vi "LabVIEW调用多模态大模型.vi"() -> ()   [LabVIEW 2023, in "LabVIEW LLM.lvlib"]
uses:
  LabVIEW LLM.lvlib
  openai_complex_message.ctl
  chat-role.ctl
  complex content.ctl
  chat-completion complex req.ctl
  <vilib>/Utility/error.llb/Trim Whitespace One-Sided.vi
  labview-ai-share/LabVIEW AI Base.lvlib
  <vilib>/JDP Science/JDP Science Common Utilities/Base64/Base64 Support.lvlib
panel:
  in  "Select Image":bool
  out "Base64 Encoded":string
  out "图片":picture
  in  "API Key":string="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"
  in  "system prompt":string caption="System提示词"
  in  "temperature (default: 0.8)":dbl=0.8 format="%.1f"
  in  "max tokens (default: 4096)":u32=4096
  in  "Clear":bool
  in  "model URL":string="https://openrouter.ai/api/v1"
  in  "Send":bool
  in  "Input":string="图片中的模块是什么型号？它有几个测量通道？能测量什么类型的信号？"
  in  "选择本地模型":string(combo)="qwen/qwen2.5-vl-3b-instruct:free"
  out "error out":errorcluster
  in  "STOP":bool
  out "对话":string
  # "LabVIEW调用多模态大模型"
  # "参数"
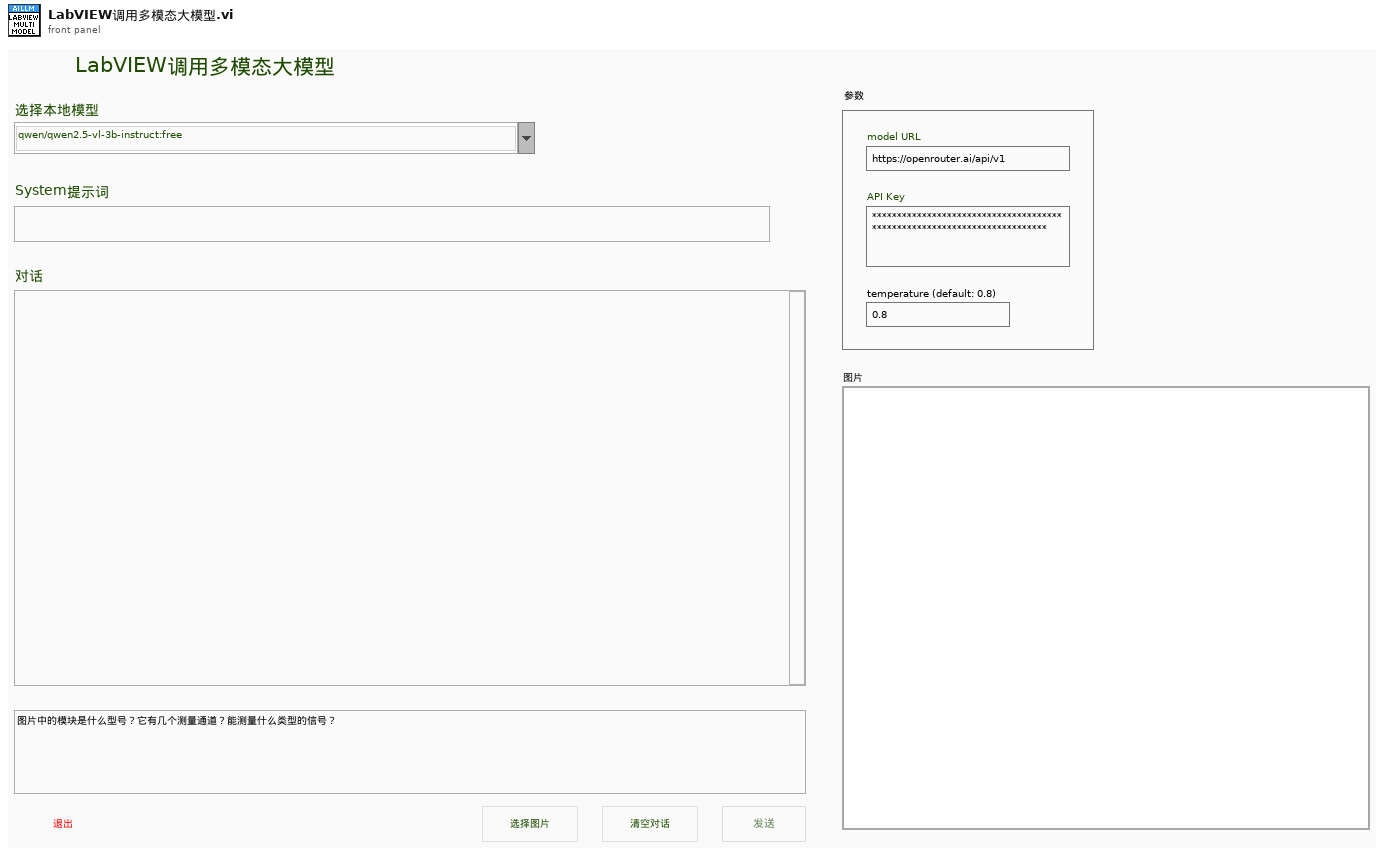
[diagram p1: front panel]
types:
  T1 = enum8{"Enabled", "Disabled", "Disabled and Grayed Out"}
  T2 = typedef "LabVIEW LLM.lvlib/openai_complex_message.ctl" = cluster{"role":T3, "content":T4[]}
  T3 = typedef "LabVIEW LLM.lvlib/chat-role.ctl" = enum16{"system", "user", "assistant"}
  T4 = typedef "LabVIEW LLM.lvlib/complex content.ctl" = cluster{"type":string, "text":string, "image_url":cluster{"url":string}}
  T5 = typedef "LabVIEWHTTPClient.lvlib/ClientHandle.ctl" = refnum<k1>
  T6 = typedef "LabVIEW LLM.lvlib/chat-completion complex req.ctl" = cluster{"model":string, "messages":T2[], "max_tokens":u32, "temperature":dbl, "stream":bool}
  T7 = typedef "LVBoundsTypeDef.ctl" = cluster{"Width":u32, "Height":u32}
  T8 = typedef "imagedata.ctl" = cluster{"image type":i32, "image depth":i32, "image":u8[], "mask":u8[], "colors":u32[], "Rectangle":cluster{"left":i16, "top":i16, "right":i16, "bottom":i16}}
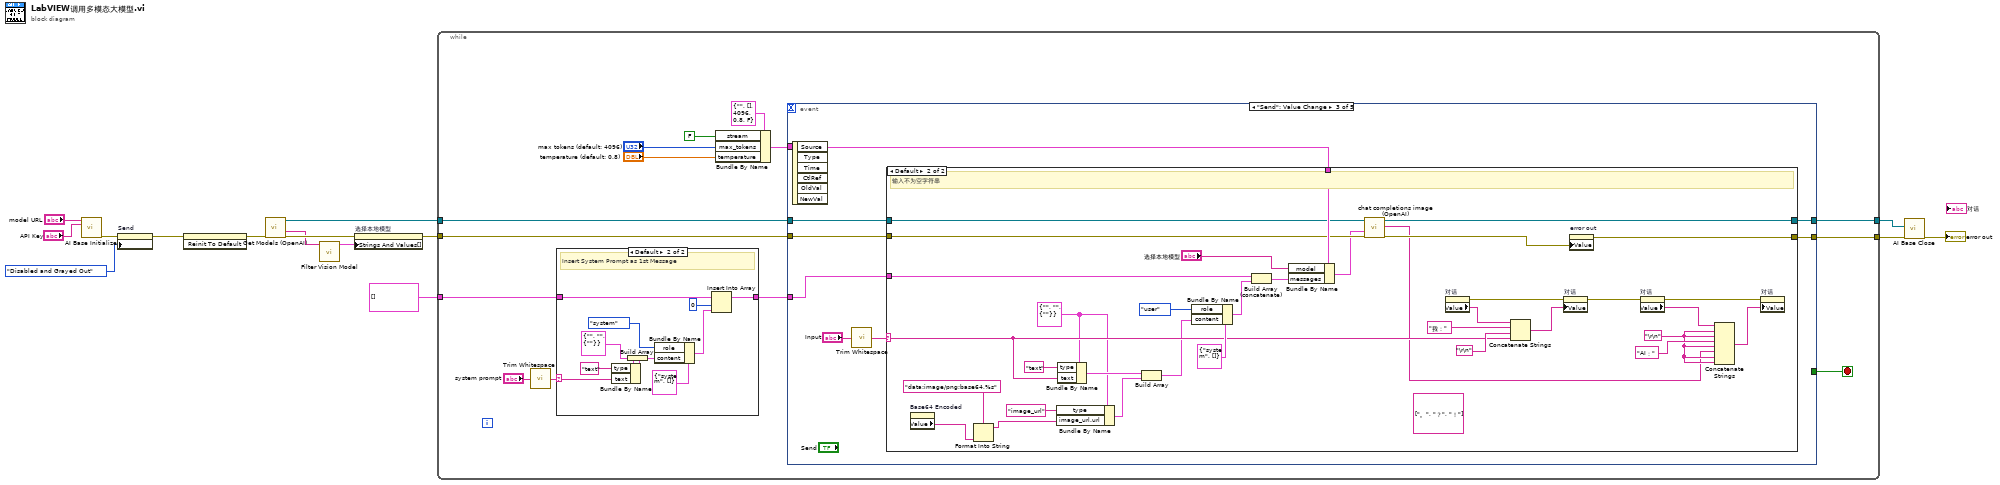
[diagram p0: block diagram]
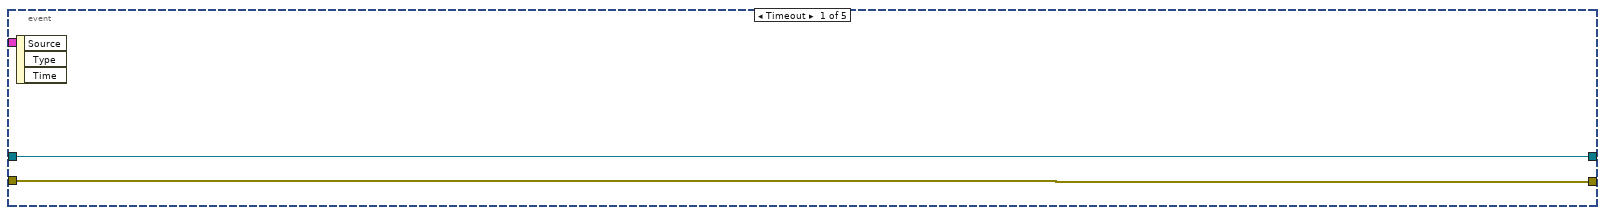
[diagram p3: hidden frame]
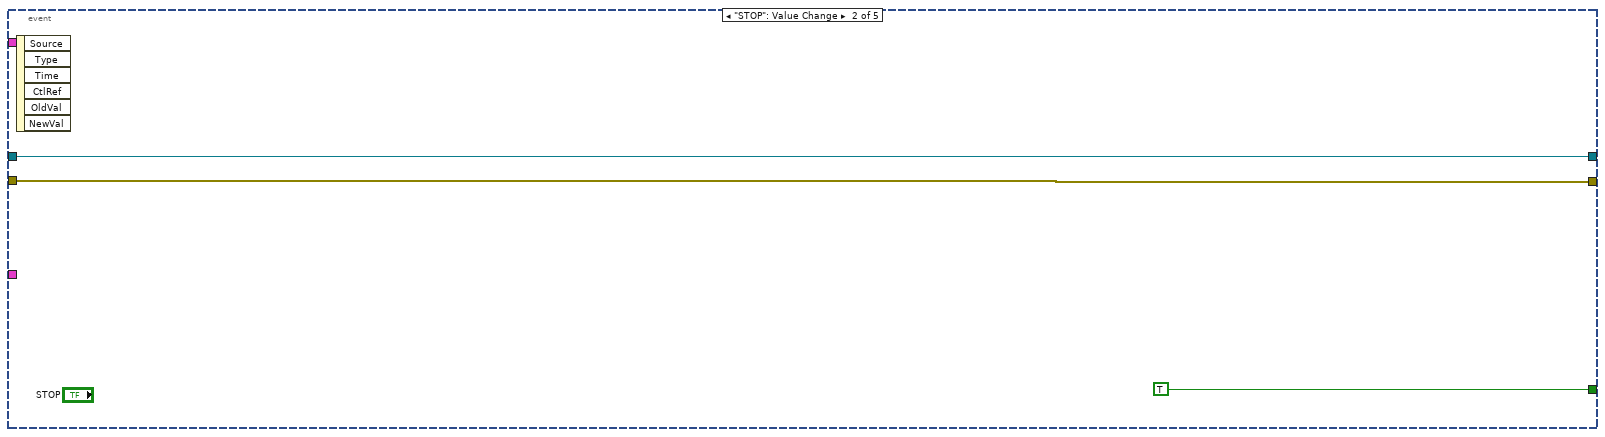
[diagram p4: hidden frame]
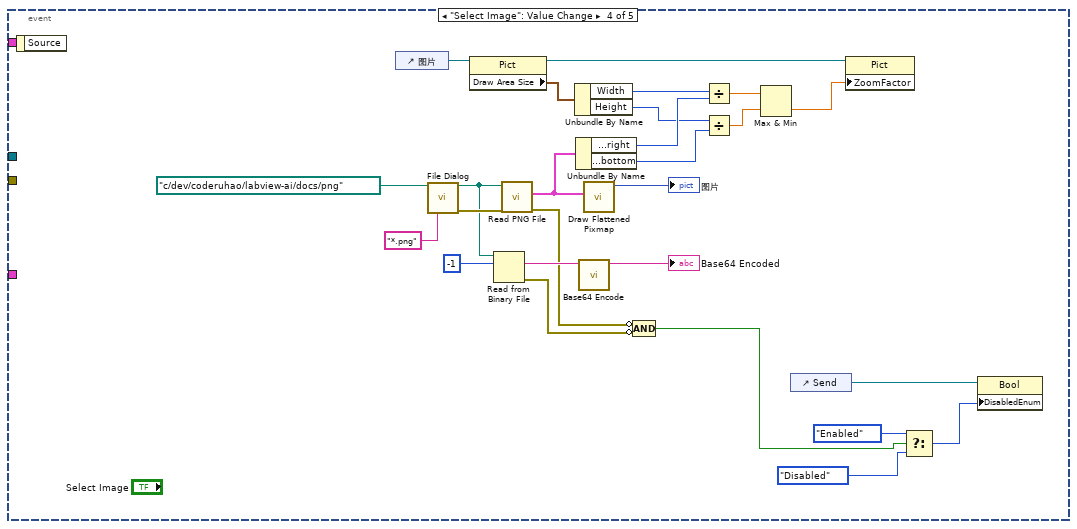
[diagram p6: hidden frame]
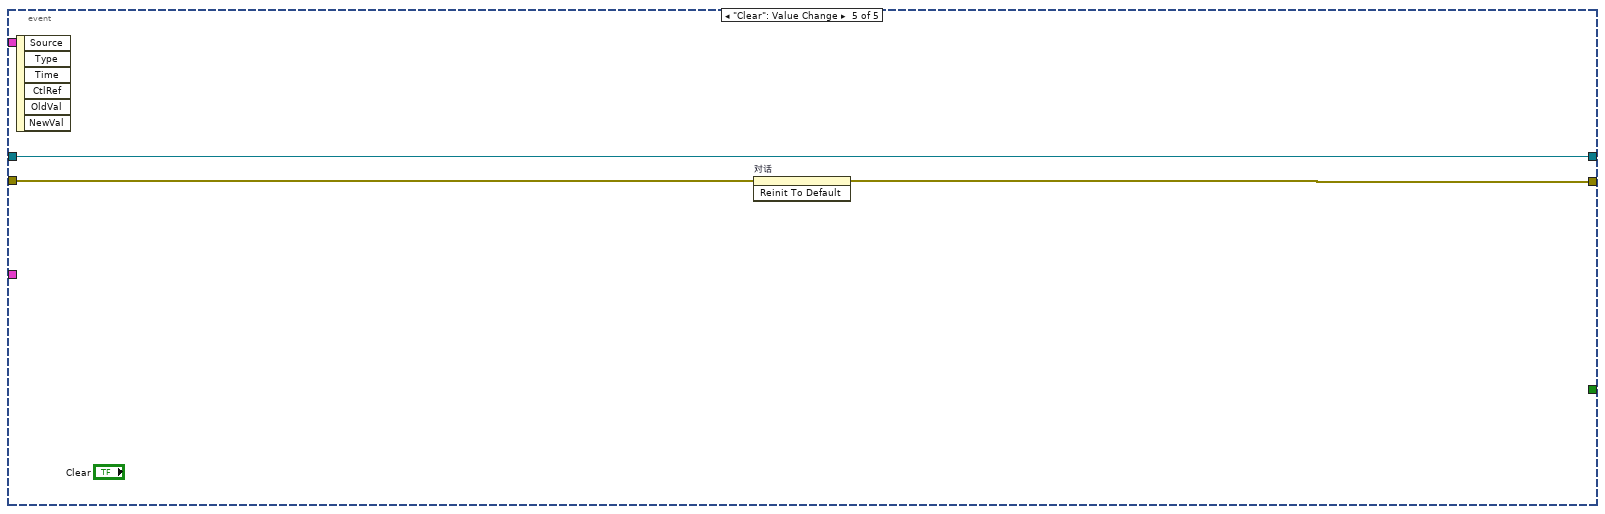
[diagram p7: hidden frame]
diagram:
  n1 = call "AI Base Initialize.vi"("OpenAI API URL"="model URL", "API Key"="API Key") -> ("error out"=w2:errorcluster)  [unwired: 11 in, 2 out]
  n2 = property on="Send" class="Bool"(error in=w2, "DisabledEnum"=T1."Disabled and Grayed Out" ("Disabled")) -> (error out=w3:errorcluster)  [unwired: 1 in, 1 out]
  n3 = invoke on="Input" class="Str" method="Reinit To Default"(error in=w3) -> (error out=w7:errorcluster)  [unwired: 2 in, 2 out]
  n4 = call "Get Models (OpenAI).vi"("error in (no error)"=w7) -> ("error out"=w10:errorcluster, "Available Models"=w8:string[], "Refnum out"=w12:T5)  [unwired: 7 in, 1 out]
  n5 = call "Filter Vision Model.vi"("Available Models"=w8) -> ("Model Rings"=w11:cluster{"String":string, "Value":string}[])  [unwired: 10 in]
  n6 = property on="选择本地模型" class="CmbBox"(error in=w10, "Strings And Values[]"=w11) -> (error out=w9:errorcluster)  [unwired: 1 in, 1 out]
  n7 = while {
    tunnel: w12 -> [w28]
    tunnel: w9 -> [w27]
    tunnel: [w26] -> w15
    tunnel: [w25] -> w14
    tunnel: T2[] [] ("previous messages") -> [w16]
    stop <- w29 stop-if-true
    n8 = call <vilib>:"Trim Whitespace.vi"("string"="system prompt") -> ("trimmed string"=w17:string)  [unwired: 1 in]
    n9 = case shown="Default" w17 {
      selector: w17 -> [_ w32]
      tunnel: w16 -> [w30 w37]
      tunnel: [w30 w39] -> w19
      frame "" {
      }
      frame Default {
        # "Insert System Prompt as 1st Message"
        n10 = Bundle By Name(cluster=T4 {"type"="", "text"="", "image_url"={"url"=""}} ("content"), "type"="text", "text"=w32) -> (w33:T4)
        n11 = Build Array(w33) -> (w34:T4[])
        n12 = Bundle By Name(cluster=T2 {"role"=enum."system", "content"=[]} ("message"), "role"=enum16{"system", "user", "assistant"}."system", "content"=w34) -> (w38:T2)
        n13 = Insert Into Array(array=w37, index=0, new element=w38) -> (w39:T2[])
      }
    }
    n14 = Bundle By Name(cluster=T6 {"model"="", "messages"=[], "max_tokens"=4096, "temperature"=0.8, "stream"=FALSE}, "stream"=FALSE ("Stream?"), "max_tokens"="max tokens (default: 4096)", "temperature"="temperature (default: 0.8)") -> (w24:T6)
    n15 = event shown="[2] \"Send\": Value Change" {
      selector: _ -> [_ _ _ _ _]
      dyn-events: _ -> [_ _ _ _ _]
      timeout: _ -> [_ _ _ _ _]
      tunnel: [_ TRUE _ _ _] -> w29
      tunnel: w28 -> [w43 w45 w51 _ w120]
      tunnel: w27 -> [w42 w44 w53 _ w119]
      tunnel: w24 -> [_ _ w54 _ _]
      tunnel: [w43 w45 w52 _ w120] -> w26
      tunnel: [w42 w44 w50 _ w118] -> w25
      tunnel: w19 -> [_ _ w48 _ _]
      event Timeout {
        n16 = event-data() -> ()  [unwired: 1 in, 3 out]
      }
      event "STOP": Value Change {
        n17 = event-data() -> ()  [unwired: 1 in, 6 out]
      }
      event "Send": Value Change {
        n18 = event-data() -> ()  [unwired: 1 in, 6 out]
        n19 = call <vilib>:"Trim Whitespace.vi"("string"="Input") -> ("trimmed string"=w47:string)  [unwired: 1 in]
        n20 = case shown="Default" w47 {
          selector: w47 -> [_ w67]
          tunnel: w54 -> [_ w91]
          tunnel: w53 -> [w56 w90]
          tunnel: [w55 w86] -> w52
          tunnel: w51 -> [w55 w85]
          tunnel: [w56 w84] -> w50
          tunnel: w48 -> [_ w71]
          frame "" {
          }
          frame Default {
            w64 = T4 {"type"="", "text"="", "image_url"={"url"=""}} ("content")
            (unwired) string[] ["。", "？", "！"] ("search string")
            w70 = "\r\n"
            # "输入不为空字符串"
            n21 = property on="Base64 Encoded" class="Str"() -> ("Value"=w62:string)  [unwired: 2 in, 2 out]
            n22 = Format Into String(format string="data:image/png;base64,%s", w62) -> (resulting string=w60:string)  [unwired: 2 in, 1 out]
            n23 = Bundle By Name(cluster=w64, "type"="image_url", "image_url.url"=w60) -> (w59:T4)
            n24 = Bundle By Name(cluster=w64, "type"="text", "text"=w67) -> (w66:T4)
            n25 = Build Array(w66, w59) -> (w65:T4[])
            n26 = Bundle By Name(cluster=T2 {"role"=enum."system", "content"=[]} ("messages"), "role"=chat-role."user", "content"=w65) -> (w58:T2)
            n27 = Build Array (concatenate)(w71, w58) -> (w87:T2[])
            n28 = Bundle By Name(cluster=w91, "model"="选择本地模型", "messages"=w87) -> (w89:T6)
            n29 = call "chat completions image (OpenAI).vi"("error in"=w90, "chat-completion req"=w89, "Refnum in"=w85) -> ("error out"=w83:errorcluster, "Answer content"=w57:string, "Refnum out"=w86:T5)  [unwired: 5 in, 1 out]
            n30 = property on="对话" class="Str"() -> (error out=w82:errorcluster, "Value"=w81:string)  [unwired: 2 in, 1 out]
            n31 = Concatenate Strings(w81, "我：" ("string"), "\r\n", w67) -> (w80:string)
            n32 = property on="对话" class="Str"(error in=w82, "Value"=w80) -> (error out=w75:errorcluster)  [unwired: 1 in, 1 out]
            n33 = property on="error out" class="Clust (strict)"("Value"=w83) -> (error out=w84:errorcluster)  [unwired: 2 in, 1 out]
            n34 = property on="对话" class="Str"(error in=w75) -> (error out=w76:errorcluster, "Value"=w73:string)  [unwired: 1 in, 1 out]
            n35 = Concatenate Strings(w73, w70, w70, "AI：" ("string"), w70, w57, w70, w70) -> (w74:string)
            n36 = property on="对话" class="Str"(error in=w76, "Value"=w74) -> ()  [unwired: 1 in, 2 out]
          }
        }
      }
      event "Select Image": Value Change {
        n37 = event-data() -> ()  [unwired: 1 in, 1 out]
        n38 = control-ref of="图片"() -> (w110:refnum<vi>)
        n39 = call "File Dialog"("start path"=path "c:/dev/coderuhao/labview-ai/docs/png", "pattern (all files)"="*.png") -> ("selected path"=w116:path, "error out"=w117:errorcluster)  [unwired: 10 in, 2 out]
        n40 = property class="Pict"(reference=w110) -> (reference out=w101:refnum<vi>, "Draw Area Size"=w108:T7)  [unwired: 1 in, 1 out]
        n41 = Read from Binary File(10:-1 ("count (1)"), 11:w116) -> (0:w96:errorcluster, 2:w115:string)  [unwired: 4 in, 2 out]
        n42 = call <vilib>:"Read PNG File.vi"("error in (no error)"=w117, "path to PNG file"=w116) -> ("error out"=w97:errorcluster, "image data"=w109:T8)  [unwired: 7 in, 1 out]
        n43 = Unbundle By Name(w108) -> ("Width"=w107:u32, "Height"=w105:u32)
        n44 = Unbundle By Name(w109) -> ("Rectangle.right"=w106:i16, "Rectangle.bottom"=w104:i16)
        n45 = call <vilib>:"Base64 Encode.vi"("String to Encode"=w115) -> ("Base64 Encoded"=→"Base64 Encoded":string)  [unwired: 10 in]
        n46 = call <vilib>:"Draw Flattened Pixmap.vi"("image data"=w109) -> ("new picture"=→"图片":picture)  [unwired: 8 in]
        n47 = Compound Arithmetic op=AND(invert w97, invert w96) -> (w93:bool)
        n48 = Divide(x=w107, y=w106) -> (x/y=w103:dbl)
        n49 = Divide(x=w105, y=w104) -> (x/y=w102:dbl)
        n50 = Max & Min(x=w103, y=w102) -> (min(x,y)=w100:dbl)  [unwired: 1 out]
        n51 = control-ref of="Send"() -> (w98:refnum<vi>)
        n52 = property class="Pict"(reference=w101, "ZoomFactor"=w100) -> ()  [unwired: 1 in, 2 out]
        n53 = Select(t=T1."Enabled" ("Disabled"), s=w93, f=T1."Disabled" ("Disabled")) -> (s? t:f=w94:T1)
        n54 = property class="Bool"(reference=w98, "DisabledEnum"=w94) -> ()  [unwired: 1 in, 2 out]
      }
      event "Clear": Value Change {
        n55 = event-data() -> ()  [unwired: 1 in, 6 out]
        n56 = invoke on="对话" class="Str" method="Reinit To Default"(error in=w119) -> (error out=w118:errorcluster)  [unwired: 2 in, 2 out]
      }
    }
  }
  n57 = call "AI Base Close.vi"("error in"=w14, "Http Refnum in"=w15) -> ("error out"=→"error out":errorcluster)  [unwired: 9 in]
